vi "Import from Project.vi"(8 "error in":errorcluster, 11 "references":T1) -> (0 "error out":errorcluster, 3 "references out":T1)   [LabVIEW 2013, in "Scan Engine editor node.lvclass"]
uses:
  Scan Engine editor node.lvclass
  <vilib>/NI/DCAF/Tag Editor Core/Table API/Table Manager/object ref.ctl
  <vilib>/NI/DCAF/Tag Editor Core/Configuration Editor/Classes/Engine Parent/Engine Parent Editor Node.lvclass
  <vilib>/NI/DCAF/Tag Editor Core/Configuration Editor/Classes/Module editor node/module editor node.lvclass
  configuration/Scan Engine configuration.lvclass
  configuration/Scan Engine configuration.lvclass/Scan Engine configuration.ctl
  <vilib>/NI/DCAF/Tag Editor Core/Configuration Editor/Classes/Module editor node/Read Module Configuration.vi
  <vilib>/NI/DCAF/Tag Editor Core/Configuration Editor/Classes/Module editor node/Write Module Configuration.vi
  <vilib>/NI/Tag Bus Module Framework/module configuration/TBM module configuration.lvclass
  <vilib>/NI/Tag Bus Module Framework/channel/TBM channel.lvclass
  <vilib>/NI/DCAF/Tag Editor Core/Table API/Table Manager/Table Manager.lvclass
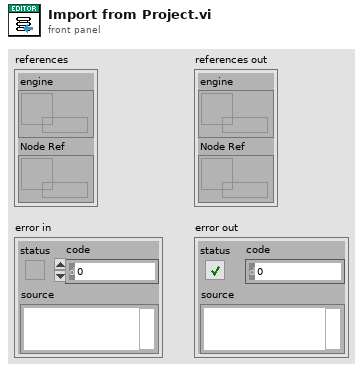
[diagram p1: front panel]
types:
  T1 = typedef "Table Manager.lvlib/Table Manager.lvclass/object ref.ctl" = cluster{"engine":refnum<data-value>, "Node Ref":refnum<data-value>}
  T2 = typedef "Scan Engine configuration.lvclass/Line.ctl" = cluster{"channel":refnum<class "TBM channel.lvclass">, "Tag":string}
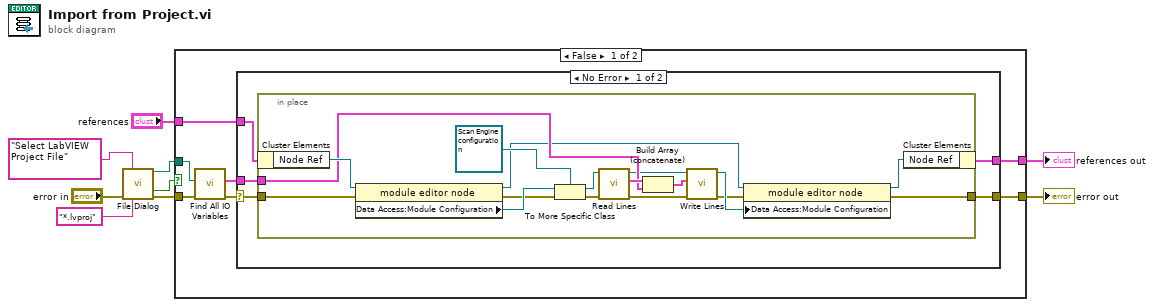
[diagram p0: block diagram]
diagram:
  n1 = call "File Dialog"("prompt"="Select LabVIEW Project File", "error in"="error in", "pattern (all files)"="*.lvproj") -> ("selected path"=w7:path, "cancelled"=w1:bool, "error out"=w3:errorcluster)  [unwired: 9 in, 1 out]
  n2 = case shown="False" w1 {
    tunnel: w7 -> [w16 _]
    tunnel: "references" -> [w14 w42]
    tunnel: [w12 w42] -> w5
    tunnel: [w11 w41] -> w4
    tunnel: w3 -> [w10 w41]
    frame False {
      n3 = call "Find All IO Variables.vi"("error in"=w10, "Path"=w16) -> ("error out"=w15:errorcluster, "Tags"=w13:T2[])  [unwired: 8 in]
      n4 = case shown="No Error" w15 {
        selector: w15 -> [w19 w39]
        tunnel: w14 -> [w21 w40]
        tunnel: w13 -> [w20 _]
        tunnel: [w18 w40] -> w12
        tunnel: [w17 w39] -> w11
        frame No Error {
          n5 = in-place {
            in-place-border: w20 -> [w33]
            in-place-border: w19 -> [w29]
            in-place-border: [w22] -> w17
            n6 = in-place-cluster #1(w21) -> ("Node Ref"=w38:refnum<data-value>)
            n7 = property class="module editor node"(reference=w38, error in=w29) -> (reference out=w28:refnum<data-value>, error out=w27:errorcluster, "Data Access:Module Configuration"=w36:refnum<class "TBM module configuration.lvclass">)
            n8 = To More Specific Class(target class=refnum<class "Scan Engine configuration.lvclass"> refnum ("Scan Engine configuration"), reference=w36, error in=w27) -> (specific class reference=w35:refnum<class "Scan Engine configuration.lvclass">, error out=w26:errorcluster)
            n9 = call "Read Lines.vi"("error in (no error)"=w26, "Scan Engine configuration in"=w35) -> ("error out"=w25:errorcluster, "Lines"=w34:T2[], "Scan Engine configuration out"=w32:refnum<class "Scan Engine configuration.lvclass">)  [unwired: 7 in]
            n10 = Build Array (concatenate)(w34, w33) -> (w31:T2[])
            n11 = call "Write Lines.vi"("error in (no error)"=w25, "Lines"=w31, "Scan Engine configuration in"=w32) -> ("error out"=w24:errorcluster, "Scan Engine configuration out"=w30:refnum<class "Scan Engine configuration.lvclass">)  [unwired: 7 in]
            n12 = property class="module editor node"(reference=w28, error in=w24, "Data Access:Module Configuration"=w30) -> (reference out=w23:refnum<data-value>, error out=w22:errorcluster)
            n13 = in-place-cluster #1("Node Ref"=w23) -> (w18:T1)
          }
        }
        frame Error {
        }
      }
    }
    frame True {
    }
  }
  "references out" <- w5
  "error out" <- w4
